vi "IsParryable.vi"(4 "User Parameter":cluster{refnum<vi>}, 5 "Event Data":cluster{"return value":bool}, 6 "Control Ref":refnum<k24>, 7 "Event Common Data":T1) -> (1 "Event Data Out":cluster{"return value":bool})   [LabVIEW 2018]
uses:
  D:/NI LabVIEW/PowerControlWithAT2/REMOTE_SEE_CONTROLLER/RemoteSeeAbleService.dll
  RemoteSeeAbleService.dll
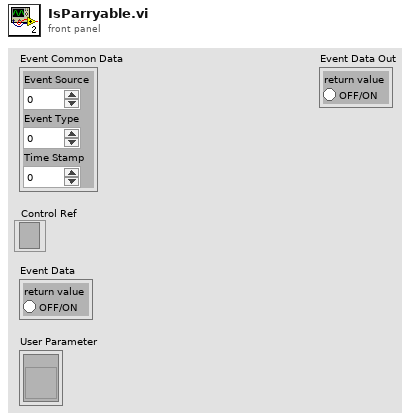
[diagram p1: front panel]
types:
  T1 = cluster{"Event Source":i32, "Event Type":u32, "Time Stamp":u32}
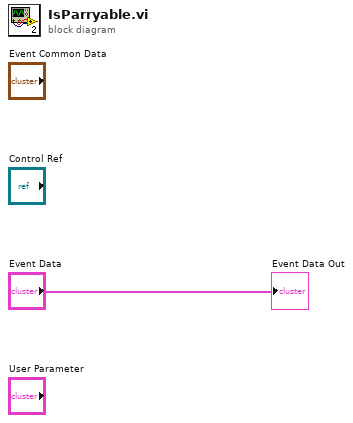
[diagram p0: block diagram]
diagram:
  "Event Data Out" <- "Event Data"
